vi "TDC_getLftHistogram.vi"(0 "Stop Channel":i32, 5 "fct in":u64, 7 "Reset":bool, 11 "Error In":errorcluster) -> (3 "Exposure Time":i64, 4 "fct out":u64, 6 "too Large":i32, 8 "Starts":i32, 10 "Stops":i32, 15 "Error Out":errorcluster)   [LabVIEW 2011]
uses:
  tdcbase.dll
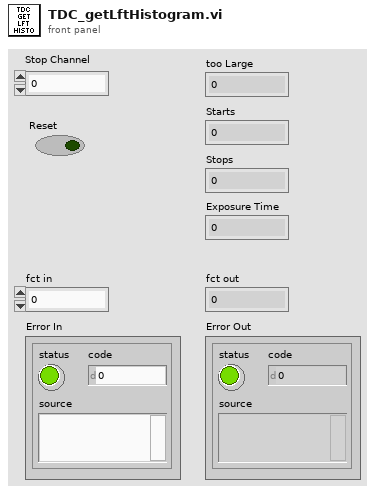
[diagram p1: front panel]
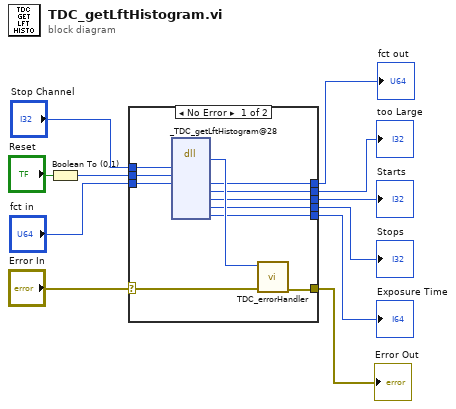
[diagram p0: block diagram]
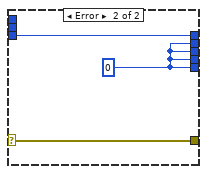
[diagram p2: hidden frame]
diagram:
  n1 = Boolean To (0,1)(Boolean="Reset") -> (0, 1=w10:i16)
  n2 = case shown="No Error" "Error In" {
    selector: "Error In" -> [w22 w25]
    tunnel: [w21 w25] -> w3
    tunnel: w10 -> [w19 _]
    tunnel: "Stop Channel" -> [w18 _]
    tunnel: [w17 w23] -> w7
    tunnel: [w16 w23] -> w6
    tunnel: [w15 w23] -> w5
    tunnel: [w14 w23] -> w4
    tunnel: "fct in" -> [w13 w24]
    tunnel: [w12 w24] -> w1
    frame No Error {
      n3 = dll-call lib="X:/tdcbase.dll" fn="_TDC_getLftHistogram@28"("channel"=w18, "reset"=w19, "fct"=w13) -> ("return type"=w20:i32, "fct"=w12:u64, "tooLarge"=w17:i32, "starts"=w16:i32, "stops"=w15:i32, "expTime"=w14:i64)  [unwired: 9 in, 2 out]
      n4 = call "TDC_errorHandler.vi"("Error In"=w22, "TDC Return Code"=w20) -> ("Error Out"=w21:errorcluster)  [unwired: 9 in]
    }
    frame Error {
      w23 = 0
    }
  }
  "too Large" <- w7
  "Stops" <- w5
  "Exposure Time" <- w4
  "Starts" <- w6
  "Error Out" <- w3
  "fct out" <- w1
